vi "Launcherdepruebas.vi"   [LabVIEW 2020]
uses:
  C:/Program Files (x86)/National Instruments/LabVIEW 2020/vi.lib/ActorFramework/Actor/Actor.lvclass
  GUI DigitalCount/GUI DigitalCount.lvclass
  <vilib>/ActorFramework/Actor/Actor.lvclass
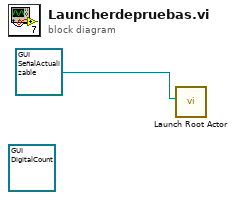
[diagram p0: block diagram]
diagram:
  (unwired) refnum<class "GUI DigitalCount.lvclass"> refnum ("GUI DigitalCount.lvlib:GUI DigitalCount.lvclass")
  n1 = call <vilib>:"Launch Root Actor.vi"("Actor"=refnum<class "GUI SeñalActualizable.lvclass"> refnum ("GUI SeñalActualizable.lvlib:GUI SeñalActualizable.lvclass")) -> ()  [unwired: 9 in, 2 out]
